vi "Initialization VI Name.vi"(11 "CD Template in":refnum<class "NIVS_PPL_Inline HW Interface.lvclass">) -> (2 "Initialization VI Name":string)   [LabVIEW 2020, in "NIVS_PPL_Inline HW Interface.lvclass"]
uses:
  NIVS_PPL_Inline HW Interface.lvclass
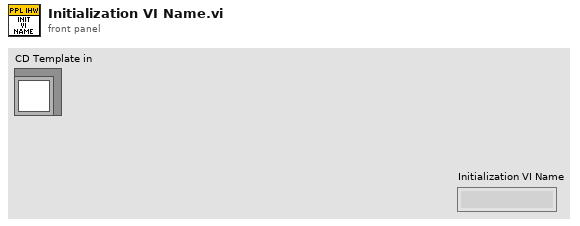
[diagram p1: front panel]
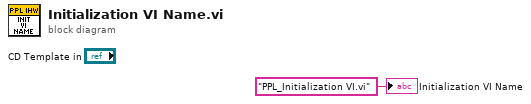
[diagram p0: block diagram]
diagram:
  "Initialization VI Name" <- "PPL_Initialization VI.vi" ("Initialization VI Name")
